vi "Center Spin Latch.vi"(11 "array":bool[](array[boolean])) -> ()   [LabVIEW 2020]
uses:
  Robot Global Data.vi
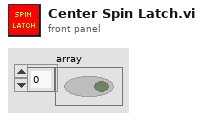
[diagram p1: front panel]
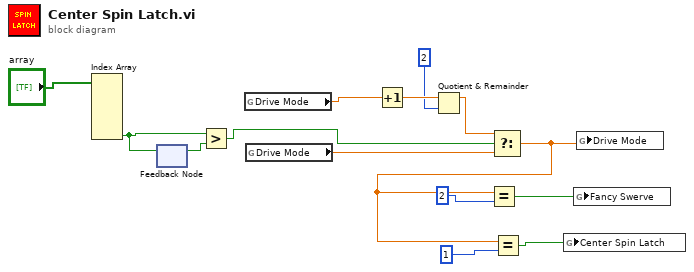
[diagram p0: block diagram]
diagram:
  n1 = Index Array(array="array") -> (element #6=w14:bool)  [unwired: 6 in, 5 out]
  n2 = feedback #1() -> (w13:bool)  [unwired: 1 in]
  n3 = feedback-in #1(w14) -> ()
  n4 = Greater?(x=w14, y=w13) -> (0:w8:bool)
  n5 = global read "Robot Global Data.vi" "Drive Mode"() -> (w11:dbl)
  n6 = global read "Robot Global Data.vi" "Drive Mode"() -> (w7:dbl)
  n7 = Increment(x=w11) -> (x+1=w10:dbl)
  n8 = Quotient & Remainder(x=w10, y=2) -> (x-y*floor(x/y)=w6:dbl)  [unwired: 1 out]
  n9 = Select(t=w6, s=w8, f=w7) -> (s? t:f=w1:dbl)
  n10 = Equal?(x=w1, y=2) -> (x = y?=w4:bool)
  n11 = Equal?(x=w1, y=1) -> (x = y?=w2:bool)
  n12 = global write "Robot Global Data.vi" "Center Spin Latch"(w2) -> ()
  n13 = global write "Robot Global Data.vi" "Fancy Swerve"(w4) -> ()
  n14 = global write "Robot Global Data.vi" "Drive Mode"(w1) -> ()
